vi "Write stop event.vi"(8 "error in (no error)":errorcluster, 10 "stop event":refnum<user-event>, 11 "Measure Object in":refnum<class "da Base.lvclass">) -> (0 "error out":errorcluster, 3 "Measure Object out":refnum<class "da Base.lvclass">)   [LabVIEW 2016, in "da Base.lvclass"]
uses:
  da Base.lvclass
  da Base.lvclass/da Base.ctl
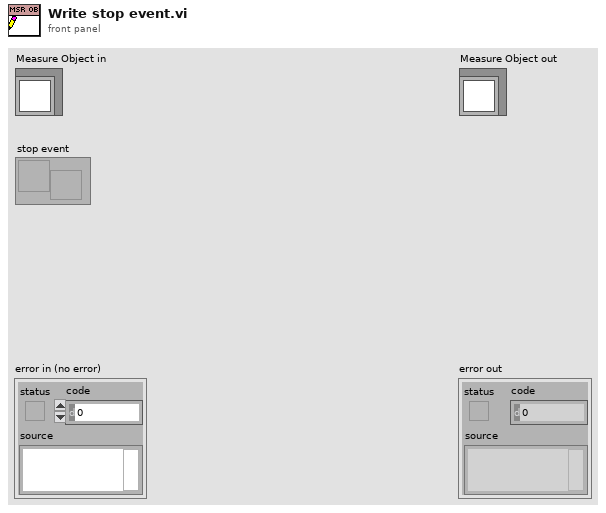
[diagram p1: front panel]
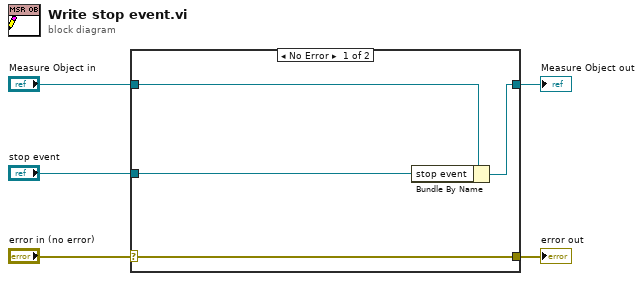
[diagram p0: block diagram]
diagram:
  n1 = case shown="No Error" "error in (no error)" {
    selector: "error in (no error)" -> [w9 w10]
    tunnel: [w9 w10] -> w4
    tunnel: [w7 w11] -> w2
    tunnel: "Measure Object in" -> [w8 w11]
    tunnel: "stop event" -> [w6 _]
    frame No Error {
      n2 = Bundle By Name(cluster=w8, "stop event"=w6) -> (w7:refnum<class "da Base.lvclass">)
    }
    frame Error {
    }
  }
  "error out" <- w4
  "Measure Object out" <- w2
